vi "Execute.vi"(8 "Error In":errorcluster, 11 "Sequencer In":refnum<class "Sequencer.lvclass">) -> (0 "Error Out":errorcluster, 3 "Sequencer Out":refnum<class "Sequencer.lvclass">)   [LabVIEW 2019, in "Sequencer.lvclass"]
uses:
  Sequencer.lvclass
  C:/Users/goo13/Documents/GIT Local/myDashBoard/Source/RT/Process/Process.lvclass
  Private/Controls/State.ctl
  Central Message Handler/Public/Controls/Message.ctl
  Process/Process.lvclass
  Central Message Handler/Central Message Handler.lvclass
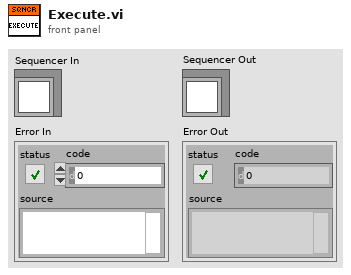
[diagram p1: front panel]
types:
  T1 = typedef "Sequencer.lvclass/State.ctl" = enum16{"Initialize", "Wait for command", "Set Dashboard", "Set Audio Analyzer", "Shutdown"}
  T2 = typedef "Central Message Handler.lvclass/Message.ctl" = cluster{"Command":string, "Data":variant, "Receiver":string}
  T3 = typedef "Process.lvclass/Process Message.ctl" = cluster{"Command":string, "Data":variant}
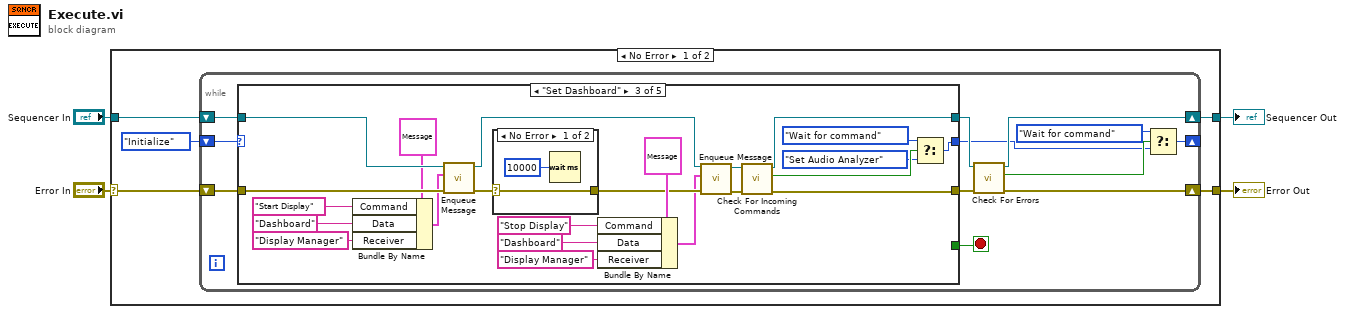
[diagram p0: block diagram]
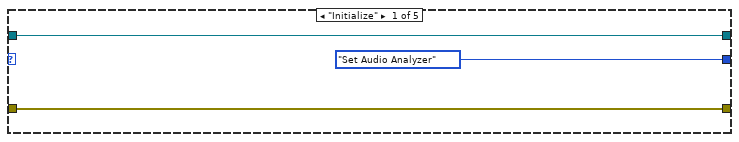
[diagram p2: hidden frame]
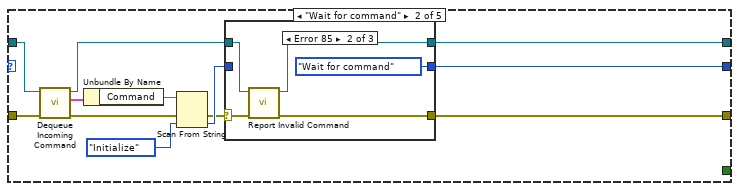
[diagram p3: hidden frame]
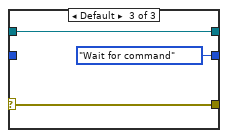
[diagram p5: hidden frame]
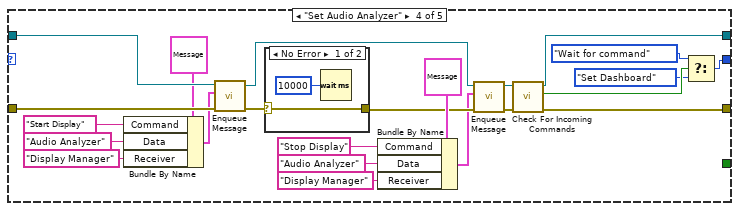
[diagram p7: hidden frame]
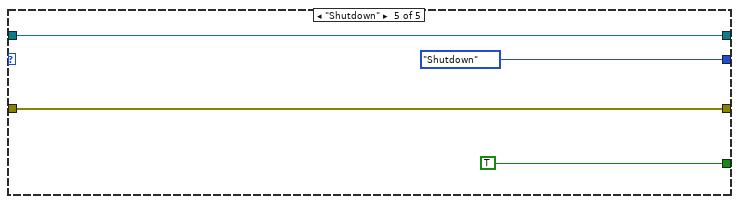
[diagram p9: hidden frame]
diagram:
  n1 = case shown="No Error" "Error In" {
    selector: "Error In" -> [w8 w105]
    tunnel: [w9 w105] -> w3
    tunnel: "Sequencer In" -> [w7 w104]
    tunnel: [w6 w104] -> w1
    frame No Error {
      n2 = while {
        shift-right: [w18] -> w9
        shift-left: w8 -> [w20]
        shift-right: [w16] -> w6
        shift-left: w7 -> [w21]
        shift-right: [w11] -> _
        shift-left: State."Initialize" ("State") -> [w15]
        stop <- w14 stop-if-true
        n3 = case shown="\"Set Dashboard\"" w15 {
          tunnel: w21 -> [w23 w35 w70 w96 w103]
          tunnel: w20 -> [w22 w36 w69 w95 w102]
          tunnel: [State."Set Audio Analyzer" ("State") w26 w57 w83 State."Shutdown" ("State")] -> w12
          tunnel: [w23 w27 w61 w87 w103] -> w17
          tunnel: [w22 w25 w58 w84 w102] -> w19
          tunnel: [_ _ _ _ TRUE] -> w14
          frame "Initialize" {
          }
          frame "Wait for command" {
            n4 = call "Dequeue Incoming Command.vi"("Error In"=w36, "Process In"=w35) -> ("Error Out"=w32:errorcluster, "Process Message"=w33:T3, "Process Out"=w34:refnum<class "Sequencer.lvclass">)  [unwired: 6 in, 1 out]
            n5 = Unbundle By Name(w33) -> ("Command"=w29:string)
            n6 = Scan From String(input string=w29, error in=w32, default 1=State."Initialize" ("State")) -> (error out=w28:errorcluster, output 1=w30:T1)  [unwired: 2 in, 2 out]
            n7 = case shown="Error 85" w28 {
              selector: w28 -> [w37 w42 w46]
              tunnel: w30 -> [w39 _ _]
              tunnel: [w39 State."Wait for command" ("State") State."Wait for command" ("State")] -> w26
              tunnel: w34 -> [w38 w44 w47]
              tunnel: [w38 w43 w47] -> w27
              tunnel: [w37 w41 w46] -> w25
              frame No Error {
              }
              frame Error {
                n8 = call "Report Invalid Command.vi"("Error In"=w42, "Process In"=w44) -> ("Error Out"=w41:errorcluster, "Process Out"=w43:refnum<class "Sequencer.lvclass">)  [unwired: 8 in]
              }
              frame Default {
              }
            }
          }
          frame "Set Dashboard" {
            n9 = Bundle By Name(cluster=T2 {"Command"="Start Display", "Data"=variant, "Receiver"="Display Manager"} ("Message"), "Command"="Start Display", "Data"="Dashboard" ("Command"), "Receiver"="Display Manager") -> (w64:T2)
            n10 = call "Enqueue Message.vi"("Error In"=w69, "Message"=w64, "Process In"=w70) -> ("Error Out"=w63:errorcluster, "Process Out"=w56:refnum<class "Sequencer.lvclass">)  [unwired: 7 in]
            n11 = case shown="No Error" w63 {
              selector: w63 -> [w71 w73]
              tunnel: [w71 w73] -> w53
              frame No Error {
                n12 = Wait (ms)(milliseconds to wait=u32 10000) -> ()  [unwired: 1 out]
              }
              frame Error {
              }
            }
            n13 = Bundle By Name(cluster=T2 {"Command"="Start Display", "Data"=variant, "Receiver"="Display Manager"} ("Message"), "Command"="Stop Display", "Data"="Dashboard" ("Command"), "Receiver"="Display Manager") -> (w52:T2)
            n14 = call "Enqueue Message.vi"("Error In"=w53, "Message"=w52, "Process In"=w56) -> ("Error Out"=w48:errorcluster, "Process Out"=w55:refnum<class "Sequencer.lvclass">)  [unwired: 7 in]
            n15 = call "Check For Incoming Commands.vi"("Error In"=w48, "Process In"=w55) -> ("Error Out"=w58:errorcluster, "New Command(s)"=w60:bool, "Process Out"=w61:refnum<class "Sequencer.lvclass">)  [unwired: 7 in]
            n16 = Select(t=State."Wait for command" ("State"), s=w60, f=State."Set Audio Analyzer") -> (s? t:f=w57:T1)
          }
          frame "Set Audio Analyzer" {
            n17 = Bundle By Name(cluster=T2 {"Command"="Start Display", "Data"=variant, "Receiver"="Display Manager"} ("Message"), "Command"="Start Display", "Data"="Audio Analyzer" ("Command"), "Receiver"="Display Manager") -> (w90:T2)
            n18 = call "Enqueue Message.vi"("Error In"=w95, "Message"=w90, "Process In"=w96) -> ("Error Out"=w89:errorcluster, "Process Out"=w80:refnum<class "Sequencer.lvclass">)  [unwired: 7 in]
            n19 = case shown="No Error" w89 {
              selector: w89 -> [w97 w99]
              tunnel: [w97 w99] -> w78
              frame No Error {
                n20 = Wait (ms)(milliseconds to wait=u32 10000) -> ()  [unwired: 1 out]
              }
              frame Error {
              }
            }
            n21 = Bundle By Name(cluster=T2 {"Command"="Start Display", "Data"=variant, "Receiver"="Display Manager"} ("Message"), "Command"="Stop Display", "Data"="Audio Analyzer" ("Command"), "Receiver"="Display Manager") -> (w77:T2)
            n22 = call "Enqueue Message.vi"("Error In"=w78, "Message"=w77, "Process In"=w80) -> ("Error Out"=w82:errorcluster, "Process Out"=w81:refnum<class "Sequencer.lvclass">)  [unwired: 7 in]
            n23 = call "Check For Incoming Commands.vi"("Error In"=w82, "Process In"=w81) -> ("Error Out"=w84:errorcluster, "New Command(s)"=w86:bool, "Process Out"=w87:refnum<class "Sequencer.lvclass">)  [unwired: 7 in]
            n24 = Select(t=State."Wait for command" ("State"), s=w86, f=State."Set Dashboard") -> (s? t:f=w83:T1)
          }
          frame "Shutdown" {
          }
        }
        n25 = call "Check For Errors.vi"("Error In"=w19, "Process In"=w17) -> ("Error Out"=w18:errorcluster, "Error Detected"=w13:bool, "Process Out"=w16:refnum<class "Sequencer.lvclass">)  [unwired: 7 in]
        n26 = Select(t=State."Wait for command", s=w13, f=w12) -> (s? t:f=w11:T1)
      }
    }
    frame Error {
    }
  }
  "Error Out" <- w3
  "Sequencer Out" <- w1
